vi "CRYWrite Config Settings.vi"(6 "error in (no error)":errorcluster, 8 "Config Data":T1) -> (0 "error out":errorcluster)   [LabVIEW 2013]
doc: "Illustrates how to create and write a configuration settings file.\n\nInstructions:\nEnter values in the controls on the front panel then click on the Run Arrow.\nTo read the file, run Read Configuration Settings File.vi located in the file\\config.llb."
uses:
  CRYMainGlobal.vi
  <vilib>/Utility/config.llb/Write Key (String).vi
  <vilib>/Utility/config.llb/NI_LVConfig.lvlib
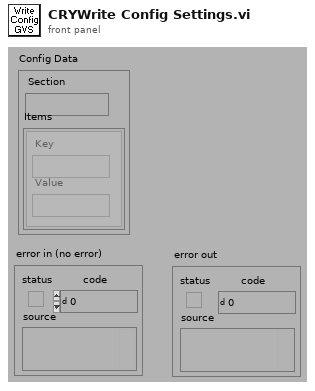
[diagram p1: front panel]
types:
  T1 = cluster{"Section":string, "Items":cluster{"Key":string, "Value":string}[]}
  T2 = typedef "NI_LVConfig.lvlib/Config Data RefNum.ctl" = refnum<k1>
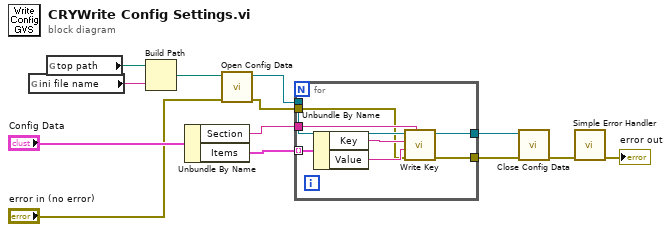
[diagram p0: block diagram]
diagram:
  n1 = global read "CRYMainGlobal.vi" "ini file name"() -> (w5:string)
  n2 = global read "CRYMainGlobal.vi" "top path"() -> (w7:path)
  n3 = Build Path(base path=w7, name or relative path=w5) -> (appended path=w4:path)
  n4 = Unbundle By Name("Config Data") -> ("Section"=w11:string, "Items"=w10:cluster{"Key":string, "Value":string}[])
  n5 = call <vilib>:"Open Config Data.vi"("error in (no error)"="error in (no error)", "configuration file path"=w4) -> ("error out"=w2:errorcluster, "refnum"=w3:T2)  [unwired: 7 in, 1 out]
  n6 = for {
    tunnel: w10 -> [w21] mode=indexing
    tunnel: w11 -> [w20]
    tunnel: [w16] -> w12
    tunnel: [w15] -> w13
    tunnel: w3 -> [w18]
    tunnel: w2 -> [w14]
    n7 = Unbundle By Name(w21) -> ("Key"=w19:string, "Value"=w17:string)
    n8 = call-poly <vilib>:"Write Key.vi"("section"=w20, "error in (no error)"=w14, "value"=w17, "key"=w19, "refnum"=w18) -> ("error out"=w15:errorcluster, "refnum out"=w16:T2)  [unwired: 1 in, 4 out]
  }
  n9 = call <vilib>:"Close Config Data.vi"("error in (no error)"=w13, "refnum"=w12) -> ("error out"=w9:errorcluster)  [unwired: 1 in, 8 out]
  n10 = call <vilib>:"Simple Error Handler.vi"("error in (no error)"=w9) -> ("error out"=→"error out":errorcluster)  [unwired: 1 in, 7 out]
